vi "Status Write starts.vi"(6 "start":bool[](array[boolean]), 8 "error in (no error)":errorcluster, 9 "Lenght (1)":i32=1, 10 "N (0)":i32, 11 "Status References":T1[](array[typedef])) -> (0 "error out":errorcluster, 3 "Status References out":T1[](array[typedef]))   [LabVIEW 2019, in "Status.lvlib"]
uses:
  Status.lvlib
  Ctl/control.ctl
  Ctl/State.ctl
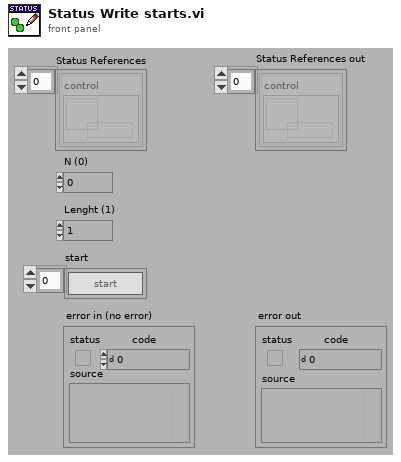
[diagram p1: front panel]
types:
  T1 = typedef "Status.lvlib/control.ctl" = cluster{"control":refnum<data-value>}
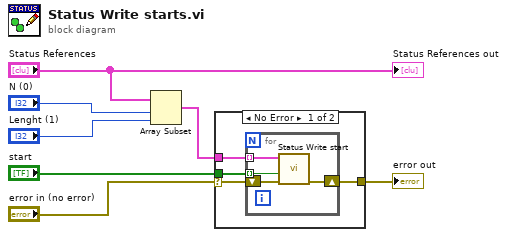
[diagram p0: block diagram]
diagram:
  n1 = Array Subset(array="Status References", index="N (0)", length="Lenght (1)") -> (w2:T1[])
  n2 = case shown="No Error" "error in (no error)" {
    selector: "error in (no error)" -> [w11 w16]
    tunnel: [w10 w16] -> w6
    tunnel: w2 -> [w9 _]
    tunnel: "start" -> [w8 _]
    frame No Error {
      n3 = for {
        shift-right: [w14] -> w10
        shift-left: w11 -> [w15]
        tunnel: w9 -> [w13] mode=indexing
        tunnel: w8 -> [w12] mode=indexing
        n4 = call "Status Write start.vi"("error in (no error)"=w15, "Start"=w12, "Status Reference"=w13) -> ("error out"=w14:errorcluster)  [unwired: 7 in, 1 out]
      }
    }
    frame Error {
    }
  }
  "error out" <- w6
  "Status References out" <- "Status References"
